vi "ClearClassNameCacheStatic.vi"(8 "error in (no error)":errorcluster, 11 "BlueSerializer in":refnum<class "BlueSerializer.lvclass">) -> (0 "error out":errorcluster, 3 "BlueSerializer out":refnum<class "BlueSerializer.lvclass">)   [LabVIEW 2019, in "BlueSerialization.lvlib" / "BlueSerializer.lvclass"]
uses:
  BlueSerializer.lvclass
  BlueSerializer.lvclass/BlueSerializer.ctl
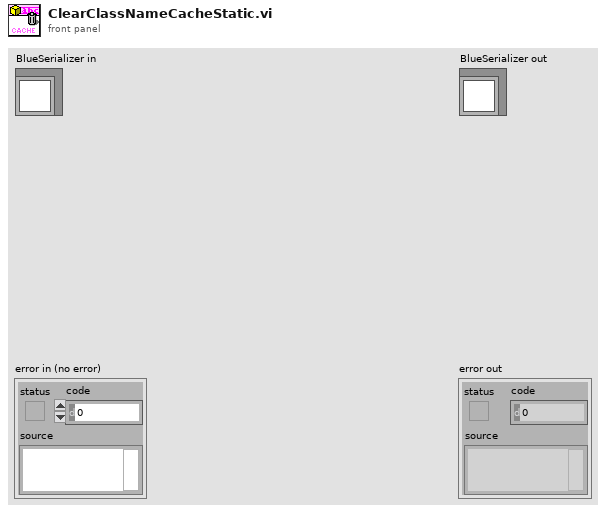
[diagram p1: front panel]
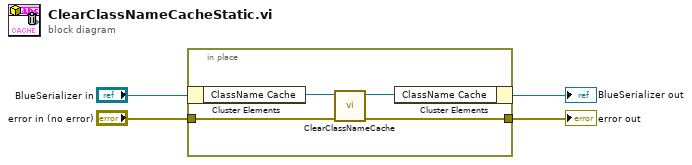
[diagram p0: block diagram]
diagram:
  n1 = in-place {
    in-place-border: "error in (no error)" -> [w8]
    in-place-border: [w7] -> w3
    n2 = in-place-cluster #1("BlueSerializer in") -> ("ClassName Cache"=w6:refnum<data-value>)
    n3 = call "ClearClassNameCache.vi"("error in (no error)"=w8, "ClassName Cache"=w6) -> ("error out"=w7:errorcluster, "ClassName Cache"=w5:refnum<data-value>)  [unwired: 8 in]
    n4 = in-place-cluster #1("ClassName Cache"=w5) -> (→"BlueSerializer out":refnum<class "BlueSerializer.lvclass">)
  }
  "error out" <- w3
